vi "Emergency Stop.vi"(8 "error in (no error)":errorcluster, 11 "Programing Logic in":refnum<class "Programing Logic.lvclass">) -> (0 "error out":errorcluster, 3 "Programing Logic out":refnum<class "Programing Logic.lvclass">)   [LabVIEW 2014, in "Programing Logic.lvclass"]
uses:
  Programing Logic.lvclass
  Programing Logic.lvclass/Programing Logic.ctl
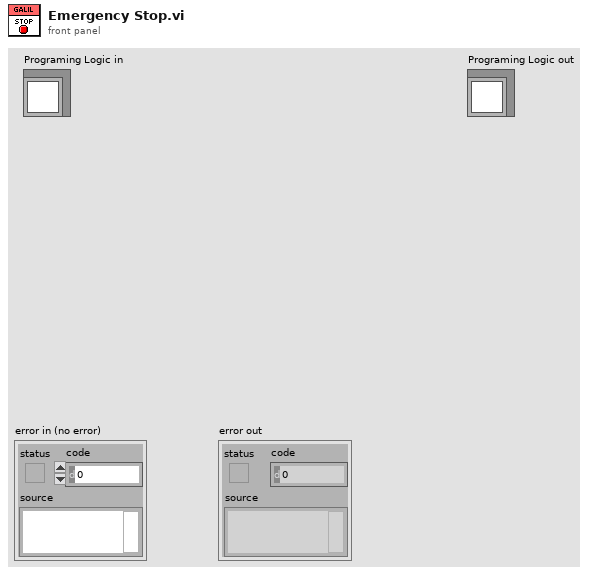
[diagram p1: front panel]
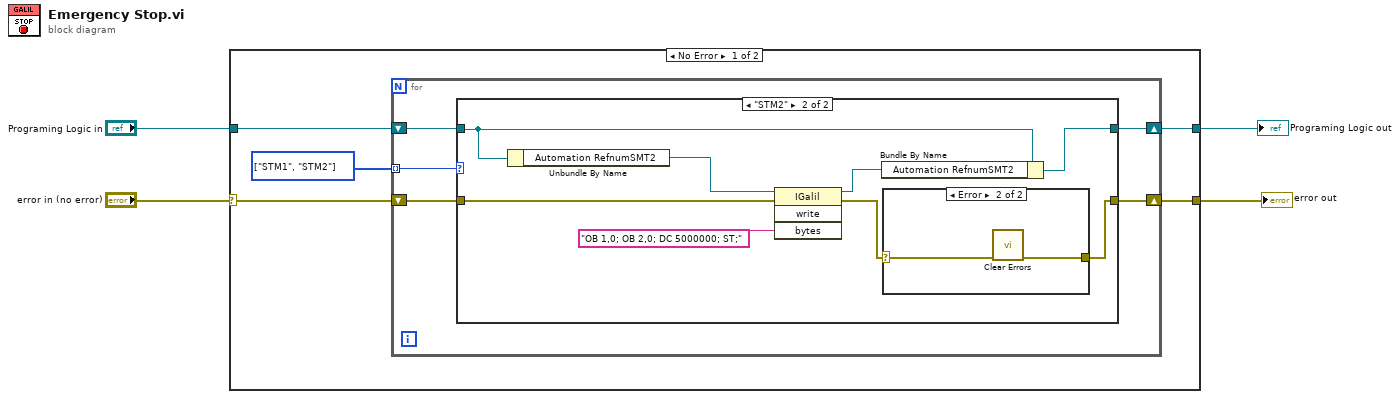
[diagram p0: block diagram]
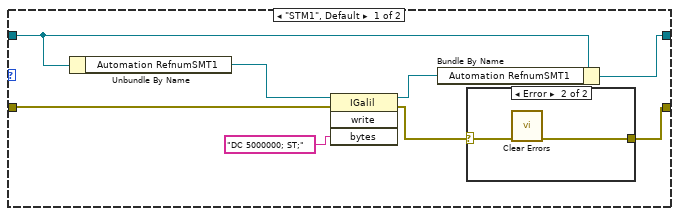
[diagram p2: hidden frame]
diagram:
  n1 = case shown="No Error" "error in (no error)" {
    selector: "error in (no error)" -> [w8 w38]
    tunnel: [w6 w38] -> w3
    tunnel: [w7 w37] -> w1
    tunnel: "Programing Logic in" -> [w9 w37]
    frame No Error {
      w5 = enum16{"STM1", "STM2", ""}[] [enum."STM1", enum."STM2"] items=["STM1", "STM2", ""]
      n2 = for {
        shift-right: [w12] -> w7
        shift-left: w9 -> [w14]
        shift-right: [w11] -> w6
        shift-left: w8 -> [w13]
        tunnel: w5 -> [w10] mode=indexing
        n3 = case shown="\"STM2\"" w10 {
          tunnel: w14 -> [w19 w32]
          tunnel: w13 -> [w20 w30]
          tunnel: [w18 w29] -> w12
          tunnel: [w15 w26] -> w11
          frame "STM1", Default {
            n4 = Unbundle By Name(w19) -> ("Automation RefnumSMT1"=w21:refnum<k7>)
            n5 = invoke class="IGalil" method="write"(reference=w21, error in=w20, "bytes"="DC 5000000; ST;") -> (reference out=w22:refnum<k7>, error out=w16:errorcluster)  [unwired: 1 in, 2 out]
            n6 = Bundle By Name(cluster=w19, "Automation RefnumSMT1"=w22) -> (w18:refnum<class "Programing Logic.lvclass">)
            n7 = case shown="Error" w16 {
              selector: w16 -> [w23 w25]
              tunnel: [w23 w24] -> w15
              frame No Error {
              }
              frame Error {
                n8 = call <vilib>:"Clear Errors.vi"("error in (no error)"=w25) -> ("error out"=w24:errorcluster)  [unwired: 5 in, 1 out]
              }
            }
          }
          frame "STM2" {
            n9 = Unbundle By Name(w32) -> ("Automation RefnumSMT2"=w33:refnum<k7>)
            n10 = invoke class="IGalil" method="write"(reference=w33, error in=w30, "bytes"="OB 1,0; OB 2,0; DC 5000000; ST;") -> (reference out=w31:refnum<k7>, error out=w27:errorcluster)  [unwired: 1 in, 2 out]
            n11 = Bundle By Name(cluster=w32, "Automation RefnumSMT2"=w31) -> (w29:refnum<class "Programing Logic.lvclass">)
            n12 = case shown="Error" w27 {
              selector: w27 -> [w34 w35]
              tunnel: [w34 w36] -> w26
              frame No Error {
              }
              frame Error {
                n13 = call <vilib>:"Clear Errors.vi"("error in (no error)"=w35) -> ("error out"=w36:errorcluster)  [unwired: 5 in, 1 out]
              }
            }
          }
        }
      }
    }
    frame Error {
    }
  }
  "error out" <- w3
  "Programing Logic out" <- w1
